vi "repmatBoolean.vi"(9 "number of repeats":dbl, 11 "Boolean":bool) -> (3 "Array":bool[](array[boolean]))   [LabVIEW 2017]
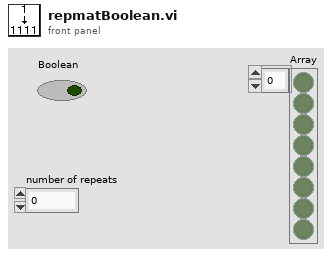
[diagram p1: front panel]
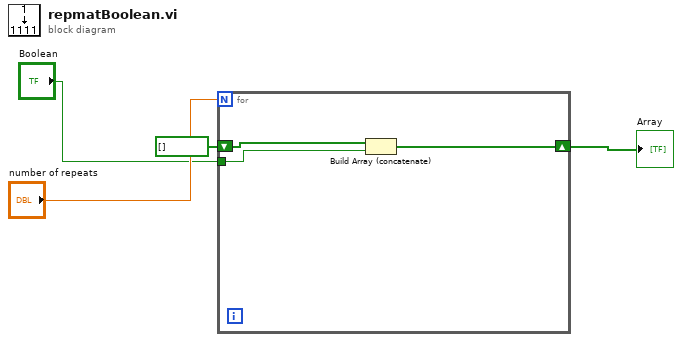
[diagram p0: block diagram]
diagram:
  n1 = for {
    N: "number of repeats" -> [_]
    tunnel: "Boolean" -> [w7]
    shift-right: [w6] -> w1
    shift-left: bool[] [] -> [w5]
    n2 = Build Array (concatenate)(w5, w7) -> (w6:bool[])
  }
  "Array" <- w1
